vi "Get Auto Focusing Status.vi"(0 "VISA Resource Name":refnum<visa-resource-name>, 5 "Device Number (1)":i32=1, 11 "error in (no error)":errorcluster {"code" format="%.0x"}) -> (4 "VISA Resource Name Out":refnum<visa-resource-name>, 6 "Status":T1(ring), 15 "error out":errorcluster {"code" format="%.0x"})   [LabVIEW 2020, in "Olympus IX BX Series.lvlib"]
doc: "Gets the focusing status of autofocusing."
uses:
  Olympus IX BX Series.lvlib
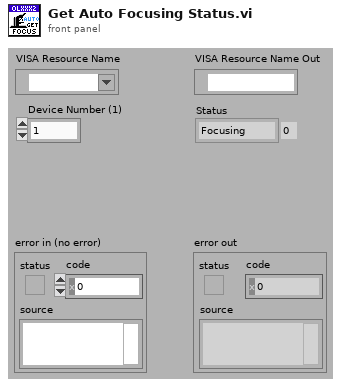
[diagram p1: front panel]
types:
  T1 = enum16{"Focusing", "Search", "Trace", "Wait", "Off"}
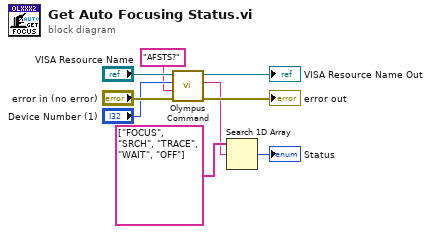
[diagram p0: block diagram]
diagram:
  n1 = call "Olympus Command.vi"("error in (no error)"="error in (no error)", "Command string"="AFSTS?" ("format string"), "Device Number (1)"="Device Number (1)", "VISA Resource Name"="VISA Resource Name") -> ("error out"=→"error out":errorcluster, "Result"=w2:string, "VISA Resource Name Out"=→"VISA Resource Name Out":refnum<visa-resource-name>)  [unwired: 5 in]
  n2 = Search 1D Array(1D array=string[] ["FOCUS", "SRCH", "TRACE", "WAIT", "OFF"], element=w2) -> (index of element=→"Status":i32)  [unwired: 1 in]
